vi "1.1nad.vi"() -> ()   [LabVIEW 2020]
uses:
  <vilib>/numeric/Random Number (Range) I64.vi
  <vilib>/numeric/sub_Random U32.vi
panel:
  out "Boolean":bool
  out "Numeric":i64
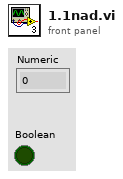
[diagram p1: front panel]
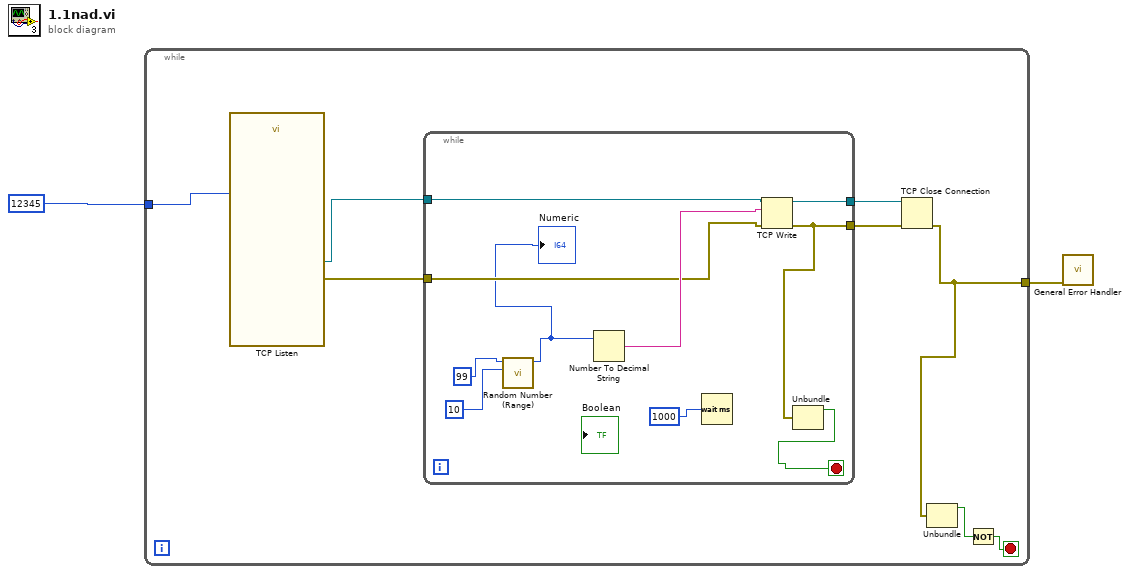
[diagram p0: block diagram]
diagram:
  n1 = while {
    tunnel: 12345 -> [w10]
    tunnel: [w5] -> w2
    stop <- w3 stop-if-true
    n2 = call <vilib>:"TCP Listen.vi"("port"=w10) -> ("error out"=w7:errorcluster, "connection ID"=w9:refnum<k5>)  [unwired: 6 in, 3 out]
    n3 = while {
      tunnel: w9 -> [w19]
      tunnel: [w20] -> w8
      tunnel: w7 -> [w17]
      tunnel: [w13] -> w6
      stop <- w11 stop-if-true
      n4 = call-poly <vilib>:"Random Number (Range).vi"("lower bound (-100)"=10, "upper bound (100)"=99) -> ("number"=w12:i64)  [unwired: 9 in]
      "Numeric" <- w12
      n5 = Number To Decimal String(number=w12) -> (decimal integer string=w18:string)  [unwired: 1 in]
      n6 = Wait (ms)(milliseconds to wait=1000) -> ()  [unwired: 1 out]
      n7 = TCP Write(connection ID=w19, data in=w18, error in (no error)=w17) -> (connection ID out=w20:refnum<k5>, error out=w13:errorcluster)  [unwired: 1 in, 1 out]
      n8 = Unbundle(w13) -> ("status"=w11:bool)  [unwired: 2 out]
    }
    n9 = TCP Close Connection(connection ID=w8, error in (no error)=w6) -> (error out=w5:errorcluster)  [unwired: 1 in, 1 out]
    n10 = Unbundle(w5) -> ("status"=w4:bool)  [unwired: 2 out]
    n11 = Not(x=w4) -> (.not. x?=w3:bool)
  }
  n12 = call <vilib>:"General Error Handler.vi"("error in (no error)"=w2) -> ()  [unwired: 10 in, 5 out]
